vi "Item Modified Timestamp.vi"(11 "Cache Item":T1) -> (3 "Modified":timestamp)   [LabVIEW 2020, in "HTTP Server.lvlib" / "Caching.lvclass"]
uses:
  Caching.lvclass
  Cache Item.ctl
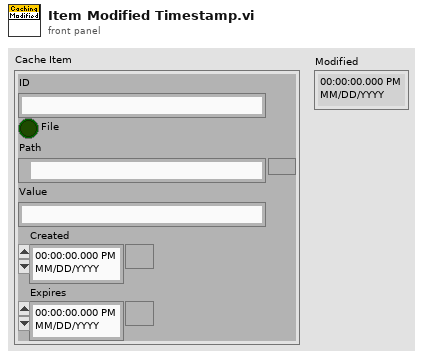
[diagram p1: front panel]
types:
  T1 = typedef "HTTP Server.lvlib/Caching.lvclass/Cache Item.ctl" = cluster{"ID":string, "File":bool, "Path":path, "Value":string, "Created":timestamp, "Expires":timestamp}
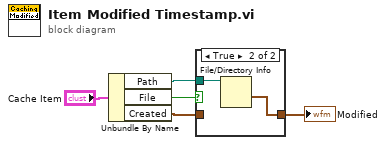
[diagram p0: block diagram]
diagram:
  n1 = Unbundle By Name("Cache Item") -> ("Path"=w3:path, "File"=w4:bool, "Created"=w2:timestamp)
  n2 = case shown="True" w4 {
    tunnel: w3 -> [_ w8]
    tunnel: w2 -> [w6 _]
    tunnel: [w6 w7] -> w1
    frame False {
    }
    frame True {
      n3 = File/Directory Info(path=w8) -> (last mod=w7:timestamp)  [unwired: 1 in, 6 out]
    }
  }
  "Modified" <- w1
